vi "Write PrefixCharacters.vi"(8 "error in (no error)":errorcluster, 10 "PrefixCharacters":string="-", 11 "ArgumentParser in":refnum<class "ArgumentParser.lvclass">) -> (0 "error out":errorcluster, 3 "ArgumentParser out":refnum<class "ArgumentParser.lvclass">)   [LabVIEW 2022 SP3, in "ArgumentParser.lvlib" / "ArgumentParser.lvclass"]
uses:
  ArgumentParser.lvclass
  ArgumentParser.lvclass/ArgumentParser.ctl
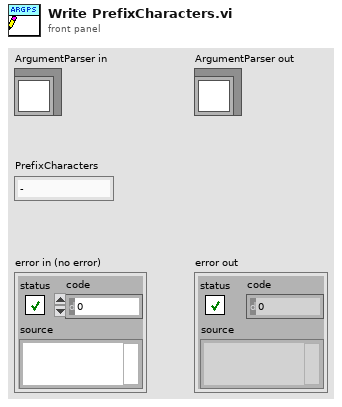
[diagram p1: front panel]
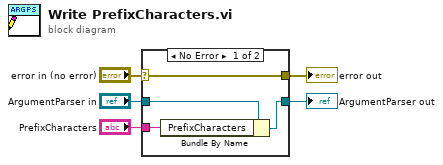
[diagram p0: block diagram]
diagram:
  n1 = case shown="No Error" "error in (no error)" {
    selector: "error in (no error)" -> [w9 w10]
    tunnel: [w9 w10] -> w4
    tunnel: [w7 w11] -> w2
    tunnel: "ArgumentParser in" -> [w8 w11]
    tunnel: "PrefixCharacters" -> [w6 _]
    frame No Error {
      n2 = Bundle By Name(cluster=w8, "PrefixCharacters"=w6) -> (w7:refnum<class "ArgumentParser.lvclass">)
    }
    frame Error {
    }
  }
  "error out" <- w4
  "ArgumentParser out" <- w2
